vi "init.vi"(8 "error in (no error)":errorcluster, 11 "ISubnet in":refnum<class "ISubnet.lvclass">) -> (0 "error out":errorcluster, 3 "ISubnet out":refnum<class "ISubnet.lvclass">)   [LabVIEW 2016, in "ISubnet.lvclass"]
uses:
  ISubnet.lvclass
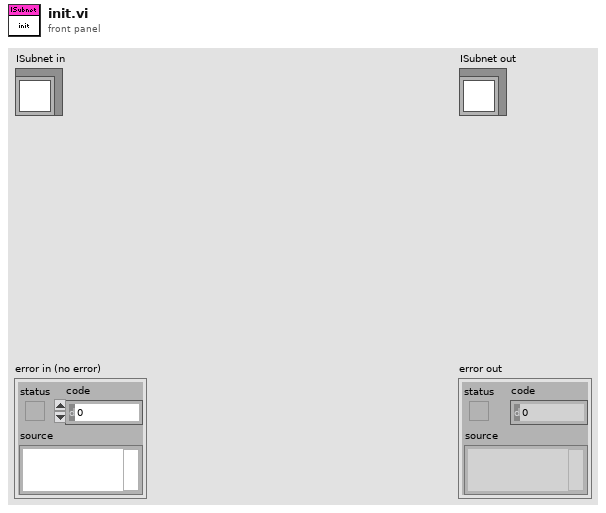
[diagram p1: front panel]
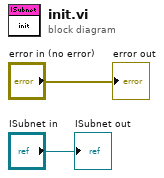
[diagram p0: block diagram]
diagram:
  "error out" <- "error in (no error)"
  "ISubnet out" <- "ISubnet in"
